vi "_io_clear_before_read.vi"(6 "Block Logging (F)":bool, 8 "error in":errorcluster caption="error in (no error)", 11 "VISA resource name":refnum<visa-resource-name>) -> (0 "error out":errorcluster, 3 "VISA resource name out":refnum<visa-resource-name>)   [LabVIEW 2020, in "Rohde&Schwarz RTx Oscilloscopes.lvlib" / "rsidr_core.lvlib"]
uses:
  rsidr_core.lvlib
  type_Error_Codes.ctl
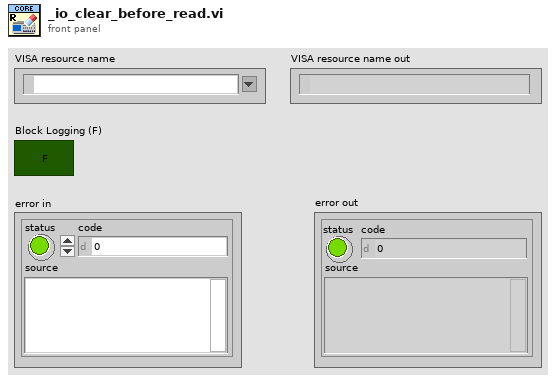
[diagram p1: front panel]
types:
  T1 = typedef "Rohde&Schwarz RTx Oscilloscopes.lvlib/rsidr_core.lvlib/type_Error_Codes.ctl" = enum16{"No_error", "VISA_err_ResourceNotFound", "VISA_err_Timeout", "VISA_warn_MoreDataAvailable", "RS_err_MissingCallback", "RS_err_InvalidAttribute", "RS_err_InvalidValue", "RS_err_UnknownResource", "RS_err_AlreadyInitialized", "RS_err_InstrumentStatus", "RS_err_BadRepCapName", "RS_err_TypesMismatch", "RS_err_ValueNotSupported", "RS_err_InvalidRngTable", "RS_err_IDqueryFail", "RS_err_UnexpResponse", "VISA_warn_ConfigNotLoaded", "RS_err_AttributeNotReadable", "RS_err_AttributeNotWritable", "RS_err_InstrumentType", "RS_err_InstrumentOption", "VISA_err_InvalidSize", "RS_err_ReliabilityIndicator", "VISA_warn_UnknownStatus", "VISA_warn_TermCharRead", "VISA_err_IO_error", "RS_err_FunctionNotSupported", "VISA_warn_QueueEmpty"}
  T2 = typedef "Rohde&Schwarz RTx Oscilloscopes.lvlib/rsidr_core.lvlib/type_Session_Data.ctl" = cluster{"IDN string":string, "Instrument FW":string, "Instr type":string, "Instr type for err. msg.":string, "Installed Options":string[], "Ignore Error Messages":string, "Logging params":variant, "OPC Timeout":i32, "VISA Timeout":i32, "STB Poll VISA Timeout":i32, "Additional Flags":i32, "Wait Before Read":i32, "Wait Before Write":i32, "Option String Flags":i32, "IO Segment Size":i64, "VISA Access Mode":T3, "Interface Type":T4, "OPC Wait Mode":T5, "Bin Float Number  Format":T6, "Bin Integer Number Format":T7, "Simulate":bool, "VXIcapable":bool, "Duplicate Session":bool, "Add LF to Write":bool, "Logging":bool, "Fast Sweep":bool, "Query Instrument Status":bool, "Check Range":bool, "Check Options":bool, "OPC-sync Attr Writes":bool, "OPC-sync Attr Queries":bool}
  T3 = typedef "Rohde&Schwarz RTx Oscilloscopes.lvlib/rsidr_core.lvlib/type_VisaAccessMode.ctl" = u16
  T4 = typedef "Rohde&Schwarz RTx Oscilloscopes.lvlib/rsidr_core.lvlib/type_InterfaceType.ctl" = enum16{"Unknown", "GPIB", "VXI", "GPIB_VXI", "ASRL", "PXI", "TCPIP", "USB", "SOCKET"}
  T5 = typedef "Rohde&Schwarz RTx Oscilloscopes.lvlib/rsidr_core.lvlib/type_OPC_Wait_Mode.ctl" = enum16{"STBpolling", "STBpollingSlow", "STBpollingSuperSlow", "ServiceRequest", "OPCquery"}
  T6 = typedef "Rohde&Schwarz RTx Oscilloscopes.lvlib/rsidr_core.lvlib/type_Binary_Float_Number_Format.ctl" = enum16{"Float_4_Bytes_Swapped", "Float_4_Bytes", "Double_8_Bytes_Swapped", "Double_8_Bytes"}
  T7 = typedef "Rohde&Schwarz RTx Oscilloscopes.lvlib/rsidr_core.lvlib/type_Binary_Integer_Number_Format.ctl" = enum16{"Int32_4_Bytes_Swapped", "Int32_4 Bytes", "Int16_2_Bytes_Swapped", "Int16_2_Bytes"}
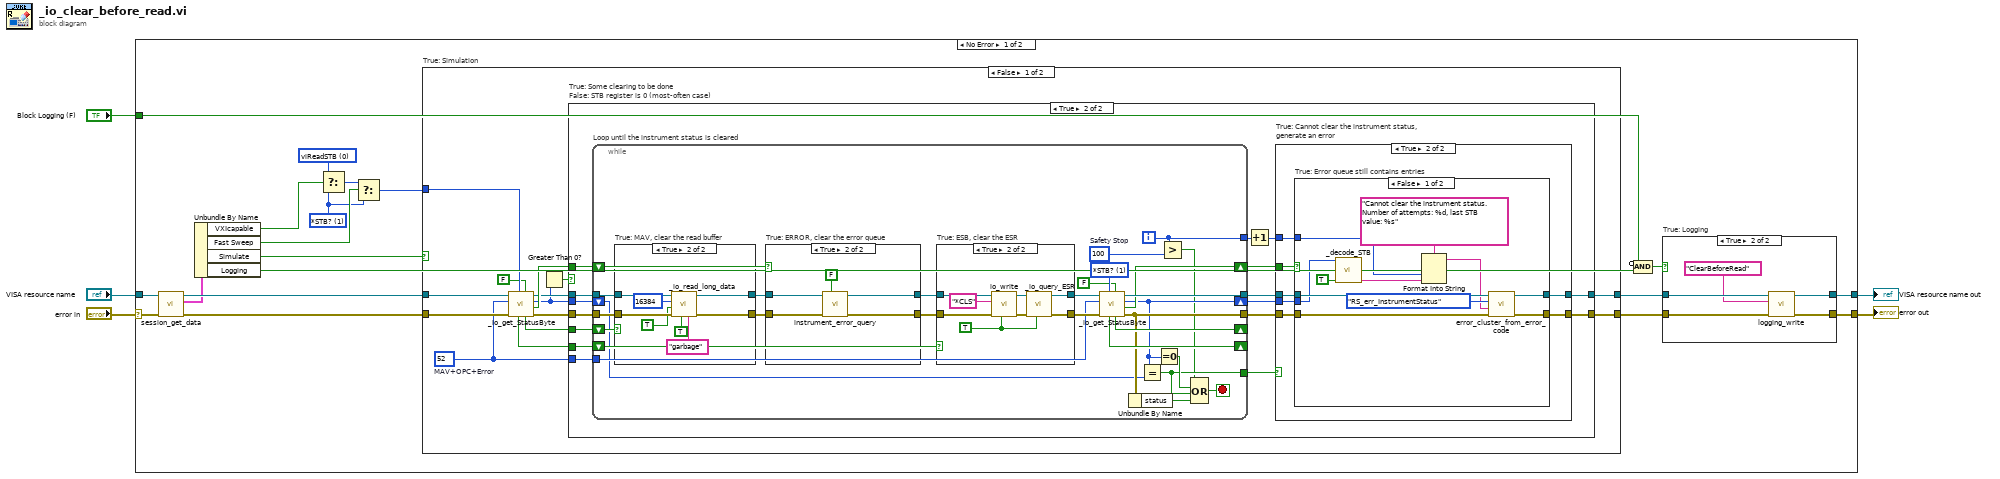
[diagram p0: block diagram]
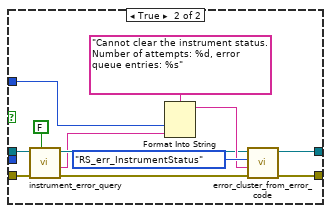
[diagram p5: hidden frame]
diagram:
  n1 = case shown="No Error" "error in" {
    selector: "error in" -> [w24 w154]
    tunnel: [w18 w154] -> w5
    tunnel: "VISA resource name" -> [w23 w153]
    tunnel: [w15 w153] -> w2
    tunnel: "Block Logging (F)" -> [w12 _]
    frame No Error {
      w11 = u16 0 items=["viReadSTB", "*STB?"] ("Method (viReadSTB)")
      w6 = u16 1 items=["viReadSTB", "*STB?"] ("Method (viReadSTB)")
      n2 = call "session_get_data.vi"("error in"=w24, "VISA resource name"=w23) -> ("error out"=w22:errorcluster, "Session User Data out"=w20:T2, "VISA resource name out"=w21:refnum<visa-resource-name>)  [unwired: 6 in, 1 out]
      n3 = Unbundle By Name(w20) -> ("VXIcapable"=w10:bool, "Fast Sweep"=w8:bool, "Simulate"=w19:bool, "Logging"=w14:bool)
      n4 = Select(t=w11, s=w10, f=w6) -> (s? t:f=w9:u16)
      n5 = Select(t=w9, s=w8, f=w6) -> (s? t:f=w7:u16)
      n6 = case "True: Simulation" shown="False" w19 {
        tunnel: [w37 w152] -> w17
        tunnel: w22 -> [w45 w152]
        tunnel: w21 -> [w44 w151]
        tunnel: [w36 w151] -> w16
        tunnel: w7 -> [w33 _]
        frame False {
          w35 = u16 52  # MAV+OPC+Error
          n7 = call "_io_get_StatusByte.vi"("Block Setting of VISA Timeout for viReadSTB"=FALSE, "Method (viReadSTB)"=w33, "error in"=w45, "Bits filter (None - 0xFF)"=w35, "VISA resource name"=w44) -> ("error out"=w39:errorcluster, "Error"=w41:bool, "STB returned"=w34:u16, "VISA resource name out"=w38:refnum<visa-resource-name>, "MAV"=w40:bool, "OPC (ESB)"=w43:bool)  [unwired: 1 in]
          n8 = Greater Than 0?(x=w34) -> (x > 0?=w42:bool)
          n9 = case "True: Some clearing to be done\nFalse: STB register is 0 (most-often case)" shown="True" w42 {
            tunnel: w39 -> [w47 w60]
            tunnel: w43 -> [_ w63]
            tunnel: w41 -> [_ w62]
            tunnel: w40 -> [_ w61]
            tunnel: w38 -> [w46 w59]
            tunnel: [w47 w54] -> w37
            tunnel: [w46 w53] -> w36
            tunnel: w35 -> [_ w58]
            tunnel: w34 -> [_ w57]
            frame False {
            }
            frame True {
              n10 = while "Loop until the instrument status is cleared" {
                tunnel: w60 -> [w121]
                shift-right: [w108] -> _
                shift-left: w63 -> [w117]
                shift-right: [w110] -> w50
                shift-left: w62 -> [w122]
                shift-right: [w109] -> _
                shift-left: w61 -> [w123]
                tunnel: w59 -> [w120]
                tunnel: [w106] -> w56
                tunnel: [w112] -> w55
                tunnel: w58 -> [w107]
                shift-right: [w104] -> w51
                shift-left: w57 -> [w105]
                tunnel: [w102] -> w52
                tunnel: [w97] -> w49
                i -> [w97]
                stop <- w100 stop-if-true
                w99 = 100  # Safety Stop
                w111 = u16 1 items=["viReadSTB", "*STB?"] ("Method (viReadSTB)")
                n11 = case "True: MAV, clear the read buffer" shown="True" w123 {
                  tunnel: w121 -> [w142 w147]
                  tunnel: w120 -> [w141 w146]
                  tunnel: [w142 w145] -> w119
                  tunnel: [w141 w144] -> w118
                  frame False {
                  }
                  frame True {
                    n12 = call "_io_read_long_data.vi"("Simulation read buffer (\"Simulation\")"="garbage" ("Simulation read buffer \n(\"Simulation\")"), "Block Logging (F)"=TRUE, "error in"=w147, "Trim Response End (T)"=TRUE, "Max segment read bytes count (65536)"=u32 16384 ("Max chunk read bytes count (65536)"), "VISA resource name"=w146) -> ("error out"=w145:errorcluster, "VISA resource name out"=w144:refnum<visa-resource-name>)  [unwired: 2 in, 2 out]
                  }
                }
                n13 = case "True: ERROR, clear the error queue" shown="True" w122 {
                  tunnel: w119 -> [w135 w139]
                  tunnel: w118 -> [w134 w140]
                  tunnel: [w135 w137] -> w116
                  tunnel: [w134 w136] -> w115
                  frame False {
                  }
                  frame True {
                    n14 = call "instrument_error_query.vi"("Add instrument error to error cluster (T)"=FALSE, "error in"=w139, "VISA resource name"=w140) -> ("error out"=w137:errorcluster, "VISA resource name out"=w136:refnum<visa-resource-name>)  [unwired: 5 in, 2 out]
                  }
                }
                n15 = case "True: ESB, clear the ESR" shown="True" w117 {
                  tunnel: w116 -> [w125 w133]
                  tunnel: w115 -> [w124 w132]
                  tunnel: [w125 w129] -> w114
                  tunnel: [w124 w128] -> w113
                  frame False {
                  }
                  frame True {
                    w127 = TRUE ("Block Logging (F)")
                    n16 = call "io_write.vi"("Block Logging (F)"=w127, "error in"=w133, "write buffer"="*CLS", "VISA resource name"=w132) -> ("error out"=w131:errorcluster, "VISA resource name out"=w130:refnum<visa-resource-name>)  [unwired: 6 in]
                    n17 = call "_io_query_ESR.vi"("Block Logging (F)"=w127, "error in"=w131, "VISA resource name"=w130) -> ("error out"=w129:errorcluster, "VISA resource name out"=w128:refnum<visa-resource-name>)  [unwired: 6 in, 1 out]
                  }
                }
                n18 = call "_io_get_StatusByte.vi"("Block Setting of VISA Timeout for viReadSTB"=FALSE, "Method (viReadSTB)"=w111, "error in"=w114, "Bits filter (None - 0xFF)"=w107, "VISA resource name"=w113) -> ("error out"=w106:errorcluster, "Error"=w110:bool, "STB returned"=w104:u16, "VISA resource name out"=w112:refnum<visa-resource-name>, "MAV"=w109:bool, "OPC (ESB)"=w108:bool)  [unwired: 1 in]
                n19 = Unbundle By Name(w106) -> ("status"=w101:bool)
                n20 = Equal?(x=w104, y=w105) -> (x = y?=w102:bool)
                n21 = Equal To 0?(x=w104) -> (x = 0?=w103:bool)
                n22 = Greater?(x=w97, y=w99) -> (0:w98:bool)
                n23 = Compound Arithmetic op=OR(w98, w103, w102, w101) -> (w100:bool)
              }
              n24 = Increment(x=w49) -> (x+1=w48:i32)
              n25 = case "True: Cannot clear the instrument status,\ngenerate an error" shown="True" w52 {
                tunnel: w56 -> [w65 w72]
                tunnel: w55 -> [w64 w71]
                tunnel: [w65 w70] -> w54
                tunnel: [w64 w69] -> w53
                tunnel: w51 -> [_ w68]
                tunnel: w50 -> [_ w66]
                tunnel: w48 -> [_ w67]
                frame False {
                }
                frame True {
                  n26 = case "True: Error queue still contains entries" shown="False" w66 {
                    tunnel: w72 -> [w83 w88]
                    tunnel: w71 -> [w82 w89]
                    tunnel: [w81 w95] -> w70
                    tunnel: [w80 w94] -> w69
                    tunnel: w68 -> [w76 _]
                    tunnel: w67 -> [w73 w90]
                    frame False {
                      n27 = call "_decode_STB.vi"("Compose Summary string (F)"=TRUE ("Compose Summary String  (F)"), "STB in"=w76) -> ("Summary string"=w74:string)  [unwired: 6 in, 3 out]
                      n28 = Format Into String(format string="Cannot clear the instrument status. Number of attempts: %d, last STB value: %s" ("error message (\"\")"), w73, w74) -> (resulting string=w77:string)  [unwired: 2 in, 1 out]
                      n29 = call "error_cluster_from_error_code.vi"("error in"=w83, "Error Message (\"\")"=w77, "Error Enum in"=type_Error_Codes."RS_err_InstrumentStatus", "VISA resource name"=w82) -> ("error out"=w81:errorcluster, "VISA resource name out"=w80:refnum<visa-resource-name>)  [unwired: 6 in]
                    }
                    frame True {
                      n30 = call "instrument_error_query.vi"("Add instrument error to error cluster (T)"=FALSE, "error in"=w88, "VISA resource name"=w89) -> ("error out"=w86:errorcluster, "Error Message(s) out"=w84:string, "VISA resource name out"=w87:refnum<visa-resource-name>)  [unwired: 5 in, 1 out]
                      n31 = Format Into String(format string="Cannot clear the instrument status. Number of attempts: %d, error queue entries: %s" ("error message (\"\")"), w90, w84) -> (resulting string=w91:string)  [unwired: 2 in, 1 out]
                      n32 = call "error_cluster_from_error_code.vi"("error in"=w86, "Error Message (\"\")"=w91, "Error Enum in"=type_Error_Codes."RS_err_InstrumentStatus", "VISA resource name"=w87) -> ("error out"=w95:errorcluster, "VISA resource name out"=w94:refnum<visa-resource-name>)  [unwired: 6 in]
                    }
                  }
                }
              }
            }
          }
        }
        frame True {
        }
      }
      n33 = Compound Arithmetic op=AND(invert w12, w14) -> (w13:bool)
      n34 = case "True: Logging" shown="True" w13 {
        tunnel: w17 -> [w26 w31]
        tunnel: [w26 w29] -> w18
        tunnel: w16 -> [w25 w30]
        tunnel: [w25 w28] -> w15
        frame False {
        }
        frame True {
          n35 = call "logging_write.vi"("error in"=w31, "String to write"="ClearBeforeRead", "VISA resource name"=w30) -> ("error out"=w29:errorcluster, "VISA resource name out"=w28:refnum<visa-resource-name>)  [unwired: 7 in]
        }
      }
    }
    frame Error {
    }
  }
  "VISA resource name out" <- w2
  "error out" <- w5
